vi "CRYGraph Property Window Digital.vi"(9 "Tab Name":string, 10 "Graph VI Ref":refnum<vi>) -> ()   [LabVIEW 2013]
panel:
  in  "Digital Tab":enum32{"Title", "Plot"}(tab)
  in  "Background Color":u32(colorbox) caption="背景颜色"
  in  "Title Name":string caption="标题名字"
  in  "OK":bool caption="UÖxÇ"
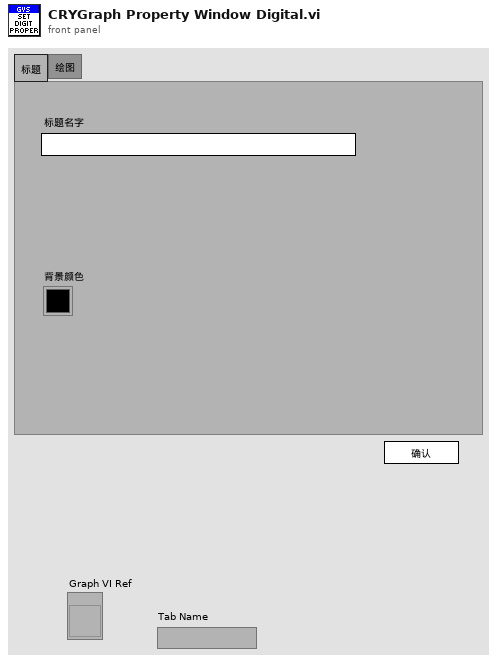
[diagram p1: front panel]
types:
  T1 = enum32{"Page Enabled", "Page Disabled", "Page Disabled & Grayed"}
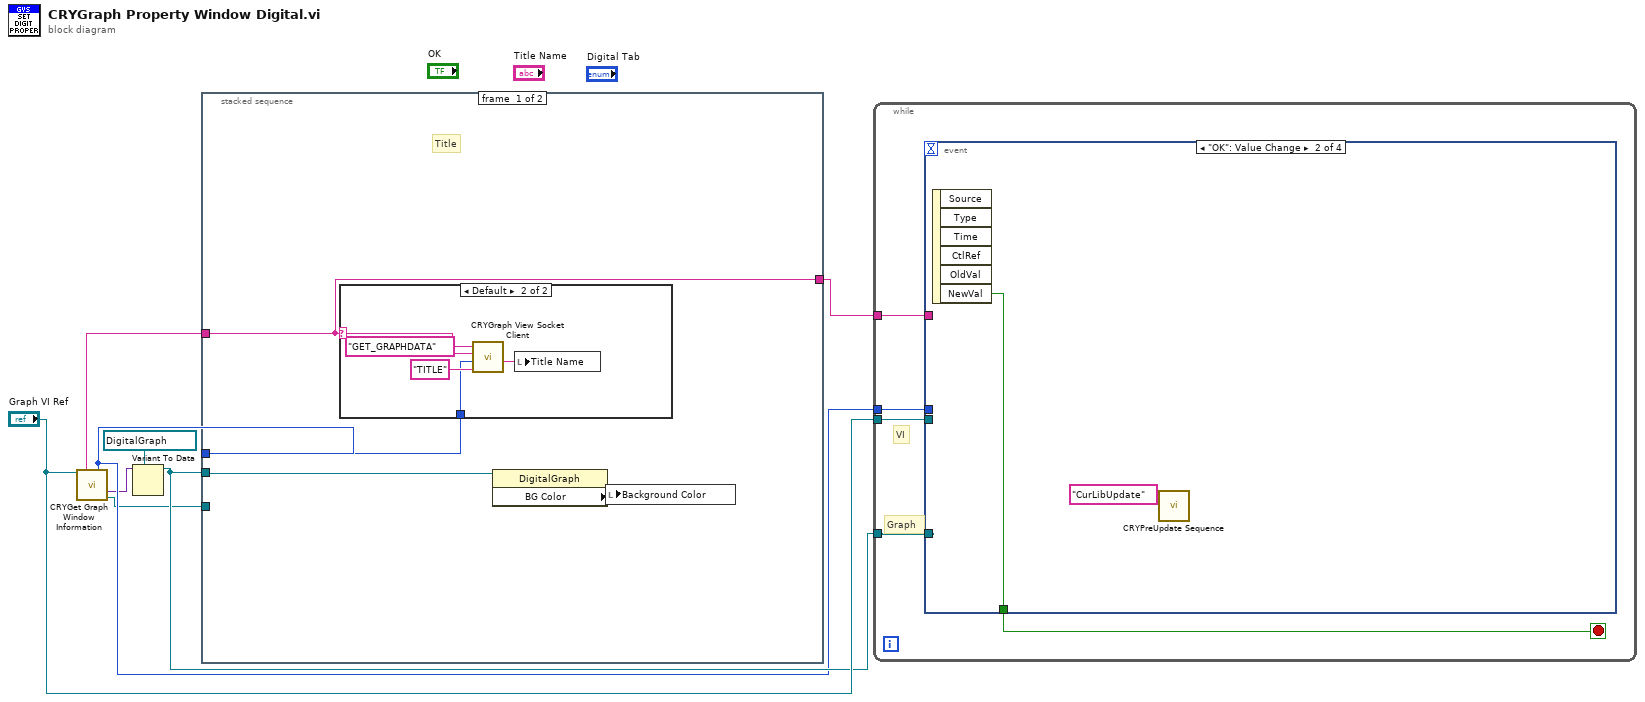
[diagram p0: block diagram]
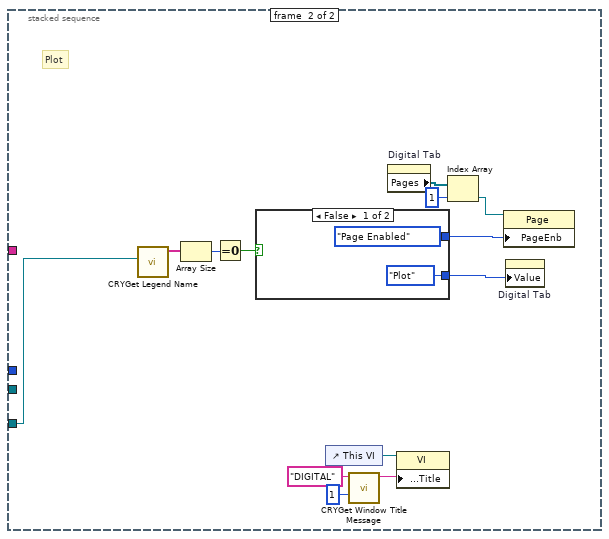
[diagram p3: hidden frame]
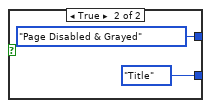
[diagram p4: hidden frame]
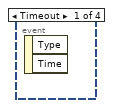
[diagram p5: hidden frame]
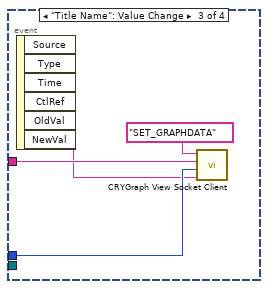
[diagram p6: hidden frame]
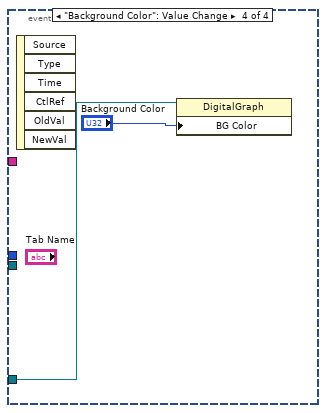
[diagram p7: hidden frame]
diagram:
  n1 = call "CRYGet Graph Window Information.vi"("pGraph VI In"="Graph VI Ref") -> ("Queue Name Out"=w5:string, "Graph Number Out"=w6:i32, "Graph Control Ref Out"=w1:variant, "Legend Ref Out"=w3:refnum<vi>)  [unwired: 4 in, 7 out]
  n2 = Variant To Data(type=refnum<vi> refnum ("Graph Ref"), Variant=w1) -> (data=w7:refnum<vi>)  [unwired: 1 in, 1 out]
  n3 = stacked-sequence {
    tunnel: w7 -> [w11 _]
    tunnel: w6 -> [w10 _]
    tunnel: w5 -> [w9 _]
    tunnel: [w9 _] -> w4
    tunnel: w3 -> [_ w22]
    frame #0 {
      # "Title"
      n4 = case shown="Default" w9 {
        selector: w9 -> [_ w14]
        tunnel: w10 -> [_ w15]
        frame "test DataView" {
        }
        frame Default {
          n5 = call "CRYGraph View Socket Client.vi"("sOption"="TITLE", "nData"=w15, "sData"=w14, "sAction"="GET_GRAPHDATA") -> ("sData Out"=w13:string)  [unwired: 4 in, 3 out]
          n6 = local write "Title Name"(w13) -> ()
        }
      }
      n7 = property class="DigitalGraph"(reference=w11) -> ("BG Color"=w12:u32)  [unwired: 1 in, 2 out]
      n8 = local write "Background Color"(w12) -> ()
    }
    frame #1 {
      # "Plot"
      n9 = call "CRYGet Legend Name.vi"("MCListbox Refnum"=w22) -> ("Names Out"=w30:string[])  [unwired: 1 in, 9 out]
      n10 = Array Size(array=w30) -> (size(s)=w29:i32)
      n11 = Equal To 0?(x=w29) -> (x = 0?=w26:bool)
      n12 = case shown="False" w26 {
        tunnel: [T1."Page Enabled" ("Page Enabled State") T1."Page Disabled & Grayed" ("Page Enabled State")] -> w24
        tunnel: [enum32{"Title", "Plot"}."Plot" ("Tab Control") enum32{"Title", "Plot"}."Title" ("Tab Control")] -> w23
        frame False {
        }
        frame True {
        }
      }
      n13 = control-ref of="This VI"() -> (w18:refnum<vi>)
      n14 = call "CRYGet Window Title Message.vi"("No"=1 ("Error No"), "Kind"="DIGITAL") -> ("Multibyte String"=w19:string)  [unwired: 4 in, 5 out]
      n15 = property on="Digital Tab" class="TabCtl (strict)"() -> ("Pages"=w28:refnum<vi>[])  [unwired: 2 in, 2 out]
      n16 = property class="VI"(reference=w18, "Front Panel.Title"=w19) -> ()  [unwired: 1 in, 2 out]
      n17 = Index Array(array=w28, index=1) -> (element=w25:refnum<vi>)
      n18 = property class="Page"(reference=w25, "PageEnb"=w24) -> ()  [unwired: 1 in, 2 out]
      n19 = property on="Digital Tab" class="TabCtl (strict)"("Value"=w23) -> ()  [unwired: 2 in, 2 out]
    }
  }
  n20 = while {
    tunnel: w7 -> [w38]
    tunnel: w6 -> [w37]
    tunnel: "Graph VI Ref" -> [w36]
    tunnel: w4 -> [w35]
    stop <- w39 stop-if-true
    # "Graph"
    # "VI"
    n21 = event shown="[1] \"OK\": Value Change" {
      selector: _ -> [_ _ _ _]
      dyn-events: _ -> [_ _ _ _]
      timeout: _ -> [_ _ _ _]
      tunnel: [_ w41 _ _] -> w39
      tunnel: w38 -> [_ _ _ w46]
      tunnel: w37 -> [_ _ w43 _]
      tunnel: w36 -> [_ _ _ _]
      tunnel: w35 -> [_ _ w44 _]
      event Timeout {
        n22 = event-data() -> ()  [unwired: 3 out]
      }
      event "OK": Value Change {
        n23 = event-data() -> ("NewVal"=w41:bool)  [unwired: 6 out]
        n24 = call "CRYPreUpdate Sequence.vi"("EventName"="CurLibUpdate") -> ()  [unwired: 15 in]
      }
      event "Title Name": Value Change {
        n25 = event-data() -> ("NewVal"=w42:string)  [unwired: 6 out]
        n26 = call "CRYGraph View Socket Client.vi"("sOption"=w42, "nData"=w43, "sData"=w44, "sAction"="SET_GRAPHDATA") -> ()  [unwired: 4 in, 4 out]
      }
      event "Background Color": Value Change {
        n27 = event-data() -> ()  [unwired: 7 out]
        n28 = property class="DigitalGraph"(reference=w46, "BG Color"="Background Color") -> ()  [unwired: 1 in, 2 out]
      }
    }
  }
